vi "View Packages and Package Attributes.vi"() -> ()   [LabVIEW 2014]
doc: "This example shows how to list installed/available/upgradable packages and view a package's attributes."
uses:
  NIPM_API.lvlib
panel:
  in  "Tab Control":T1(tab)
  out "Installed packages":string[][](table)
  out "Available packages to install":string[][](table)
  out "Upgradable packages":string[](array[string])
  in  "List packages?":bool
  in  "Get package attributes?":bool
  in  "Package name":string
  in  "Version":string
  out "Package Attributes":string[][](table)
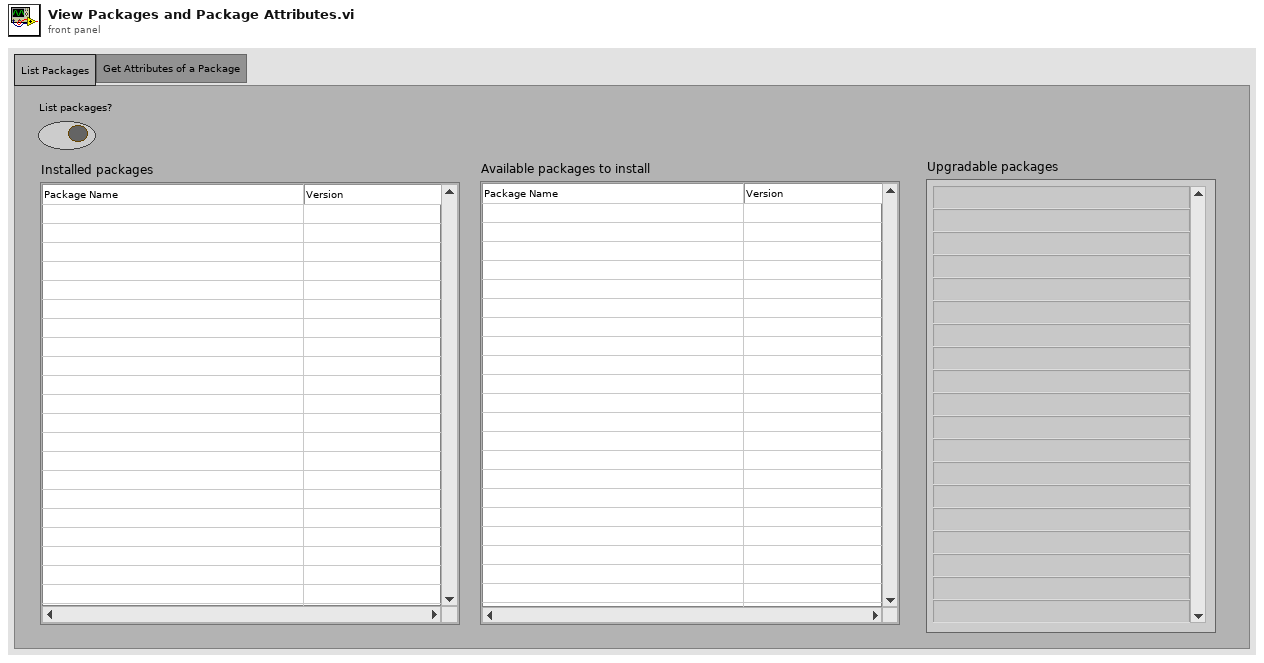
[diagram p1: front panel]
types:
  T1 = enum32{"List Packages", "Get Attributes of a Package"}
  T2 = typedef "NIPM_API.lvlib/package attributes.ctl" = cluster{"Package Name":string, "Display name":string, "Version":string, "Display version":string, "Synopsis":string, "Description":string, "Maintainer":string, "Maintainer email address":string, "Category":string, "Homepage":string, "Release notes":string, "Depends":string[], "Recommends":string[], "Suggests":string[], "Conflicts":string[], "Provides":string[], "Replaces":string[], "Supplements":string[], "Enhances":string[], "Product":bool, "User visible":bool, "Installed size (KB)":u64, "Package filesize (bytes)":u64, "Architecture":string, "Agent":string, "MD5Checksum":string}
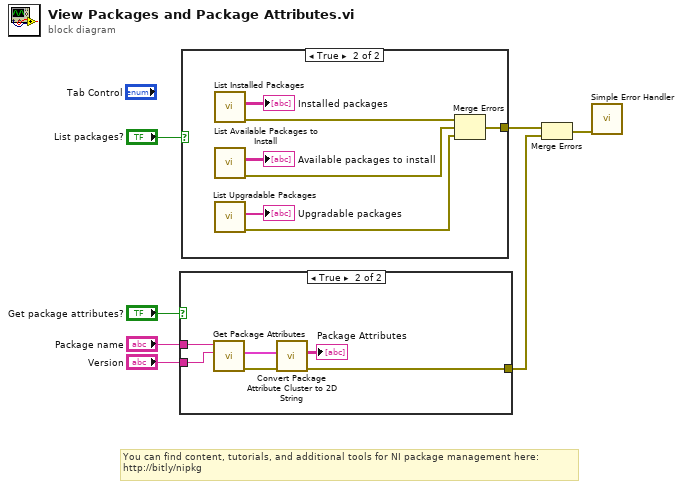
[diagram p0: block diagram]
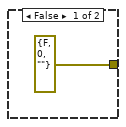
[diagram p2: hidden frame]
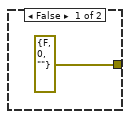
[diagram p3: hidden frame]
diagram:
  # "You can find content, tutorials, and additional tools for NI package management here:\nhttp://bitly/nipkg"
  n1 = case shown="True" "Get package attributes?" {
    tunnel: "Package name" -> [_ w14]
    tunnel: "Version" -> [_ w13]
    tunnel: [errorcluster {"status"=FALSE, "code"=0, "source"=""} ("error IO") w9] -> w1
    frame False {
    }
    frame True {
      n2 = call "Get Package Attributes.vi"("version"=w13, "package name"=w14) -> ("error out"=w11:errorcluster, "package attributes"=w12:T2)  [unwired: 6 in, 2 out]
      n3 = call "Convert Package Attribute Cluster to 2D String.vi"("error in (no error)"=w11, "package attributes (cluster)"=w12) -> ("error out"=w9:errorcluster, "package attributes (2D string)"=→"Package Attributes":string[][])  [unwired: 8 in]
    }
  }
  n4 = case shown="True" "List packages?" {
    tunnel: [errorcluster {"status"=FALSE, "code"=0, "source"=""} ("error IO") w16] -> w2
    frame False {
    }
    frame True {
      n5 = call "List Installed Packages.vi"() -> ("error out"=w19:errorcluster, "installed packages"=→"Installed packages":string[][])  [unwired: 10 in]
      n6 = call "List Available Packages to Install.vi"() -> ("error out"=w18:errorcluster, "available packages to install"=→"Available packages to install":string[][])  [unwired: 10 in]
      n7 = call "List Upgradable Packages.vi"() -> ("error out"=w17:errorcluster, "upgradable packages"=→"Upgradable packages":string[])  [unwired: 10 in]
      n8 = Merge Errors(w19, w18, w17) -> (w16:errorcluster)
    }
  }
  n9 = Merge Errors(w2, w1) -> (w3:errorcluster)
  n10 = call <vilib>:"Simple Error Handler.vi"("error in (no error)"=w3) -> ()  [unwired: 4 in, 5 out]
